vi "UI.vi"(8 "error in (no error)":errorcluster, 11 "View in":refnum<class "View.lvclass">) -> (0 "error out":errorcluster, 3 "View out":refnum<class "View.lvclass">)   [LabVIEW 2024, in "GUI.lvlib" / "View.lvclass"]
uses:
  View.lvclass
  Buttons/ButtonWhite.ctl
  Buttons/ButtonBlack.ctl
  Buttons/Key.ctl
  Buttons/Backspace.ctl
  Buttons/EnterKey.ctl
  TypeDefs/Yellow.ctl
  TypeDefs/Green.ctl
  TypeDefs/Grey.ctl
  TypeDefs/Red.ctl
  TypeDefs/White.ctl
  TypeDefs/LightGrey.ctl
  View.lvclass/View.ctl
panel:
  in  "Tab Control":enum32{"Home", "Settings", "Game", "Scores"}(tab)
  in  "Start Button":T1
  in  "Settings Button":T2
  in  "Back Button":T1
  in  "Difficulty":i32(slide)=1 min=1 max=5 step=1 scale=1.0..5.0
  in  "Guess Board":T3
  in  "Keyboard":T7
  in  "Home Button":T1
  in  "High Scores":i32(listbox)
  # "Easy"
  # "Hard"
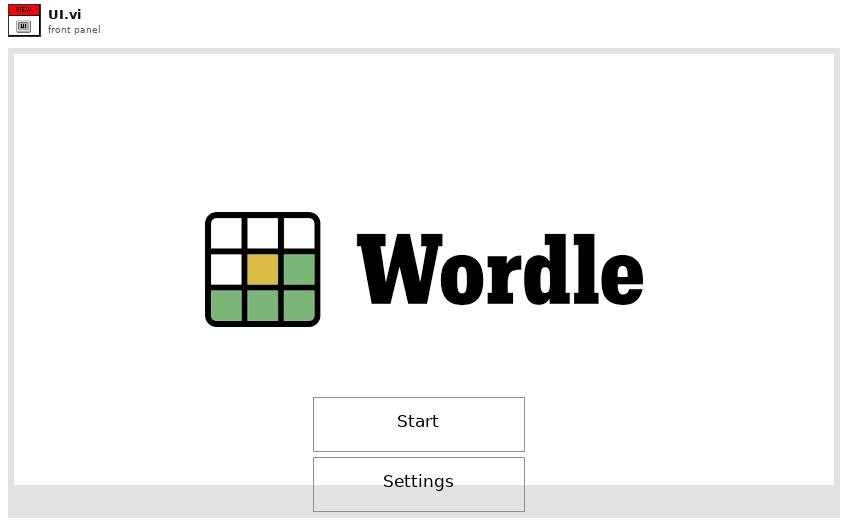
[diagram p1: front panel]
types:
  T1 = typedef "ButtonBlack.ctl" = bool
  T2 = typedef "ButtonWhite.ctl" = bool
  T3 = cluster{"Guess 1":cluster{"Letter 1":string, "Letter 2":string, "Letter 3":string, "Letter 4":string, "Letter 5":string}, "Guess 2":cluster{"Letter 1":string, "Letter 2":string, "Letter 3":string, "Letter 4":string, "Letter 5":string}, "Guess 3":cluster{"Letter 1":string, "Letter 2":string, "Letter 3":string, "Letter 4":string, "Letter 5":string}, "Guess 4":cluster{"Letter 1":string, "Letter 2":string, "Letter 3":string, "Letter 4":string, "Letter 5":string}, "Guess 5":cluster{"Letter 1":string, "Letter 2":string, "Letter 3":string, "Letter 4":string, "Letter 5":string}, "Guess 6":cluster{"Letter 1":string, "Letter 2":string, "Letter 3":string, "Letter 4":string, "Letter 5":string}}
  T4 = typedef "Key.ctl" = bool
  T5 = typedef "Backspace.ctl" = bool
  T6 = typedef "EnterKey.ctl" = bool
  T7 = cluster{"Q":T4, "W":T4, "E":T4, "R":T4, "T":T4, "Y":T4, "U":T4, "I":T4, "O":T4, "P":T4, "A":T4, "S":T4, "D":T4, "F":T4, "G":T4, "H":T4, "J":T4, "K":T4, "L":T4, "Z":T4, "X":T4, "C":T4, "V":T4, "B":T4, "N":T4, "M":T4, "Backspace":T5, "Enter":T6}
  T8 = typedef "LightGrey.ctl" = u32
  T9 = typedef "White.ctl" = u32
  T10 = typedef "Red.ctl" = u32
  T11 = typedef "Grey.ctl" = u32
  T12 = typedef "Green.ctl" = u32
  T13 = typedef "Yellow.ctl" = u32
  T14 = cluster{"This VI":refnum<vi>, "Tab Control":refnum<vi>, "Start Button":refnum<vi>, "Settings Button":refnum<vi>, "Back Button":refnum<vi>, "Difficulty":refnum<vi>, "Guess Board":refnum<vi>, "Keyboard":refnum<vi>, "High Scores":refnum<vi>, "Home Button":refnum<vi>}
  T15 = typedef "eventvkey.ctl" = enum16{"ASCII", "Enter", "Return", "Shift", "Ctrl", "Alt", "Cmd", "Opt", "Caps", "NumLock", "Clear", "Break", "Up", "Down", "Left", "Right", "Insert", "Delete", "Home", "End", "PageUp", "PageDown", "Escape", "Help", "Pause", "ScrollLock", "F1", "F2", "F3", "F4", "F5", "F6", "F7", "F8", "F9", "F10", "F11", "F12", "F13", "F14", "F15", "F16", "F17", "F18", "F19", "F20", "F21", "F22", "F23", "F24", "Play", "VolumeUp", "VolumeDown", "Mute", "Two Byte Char"}
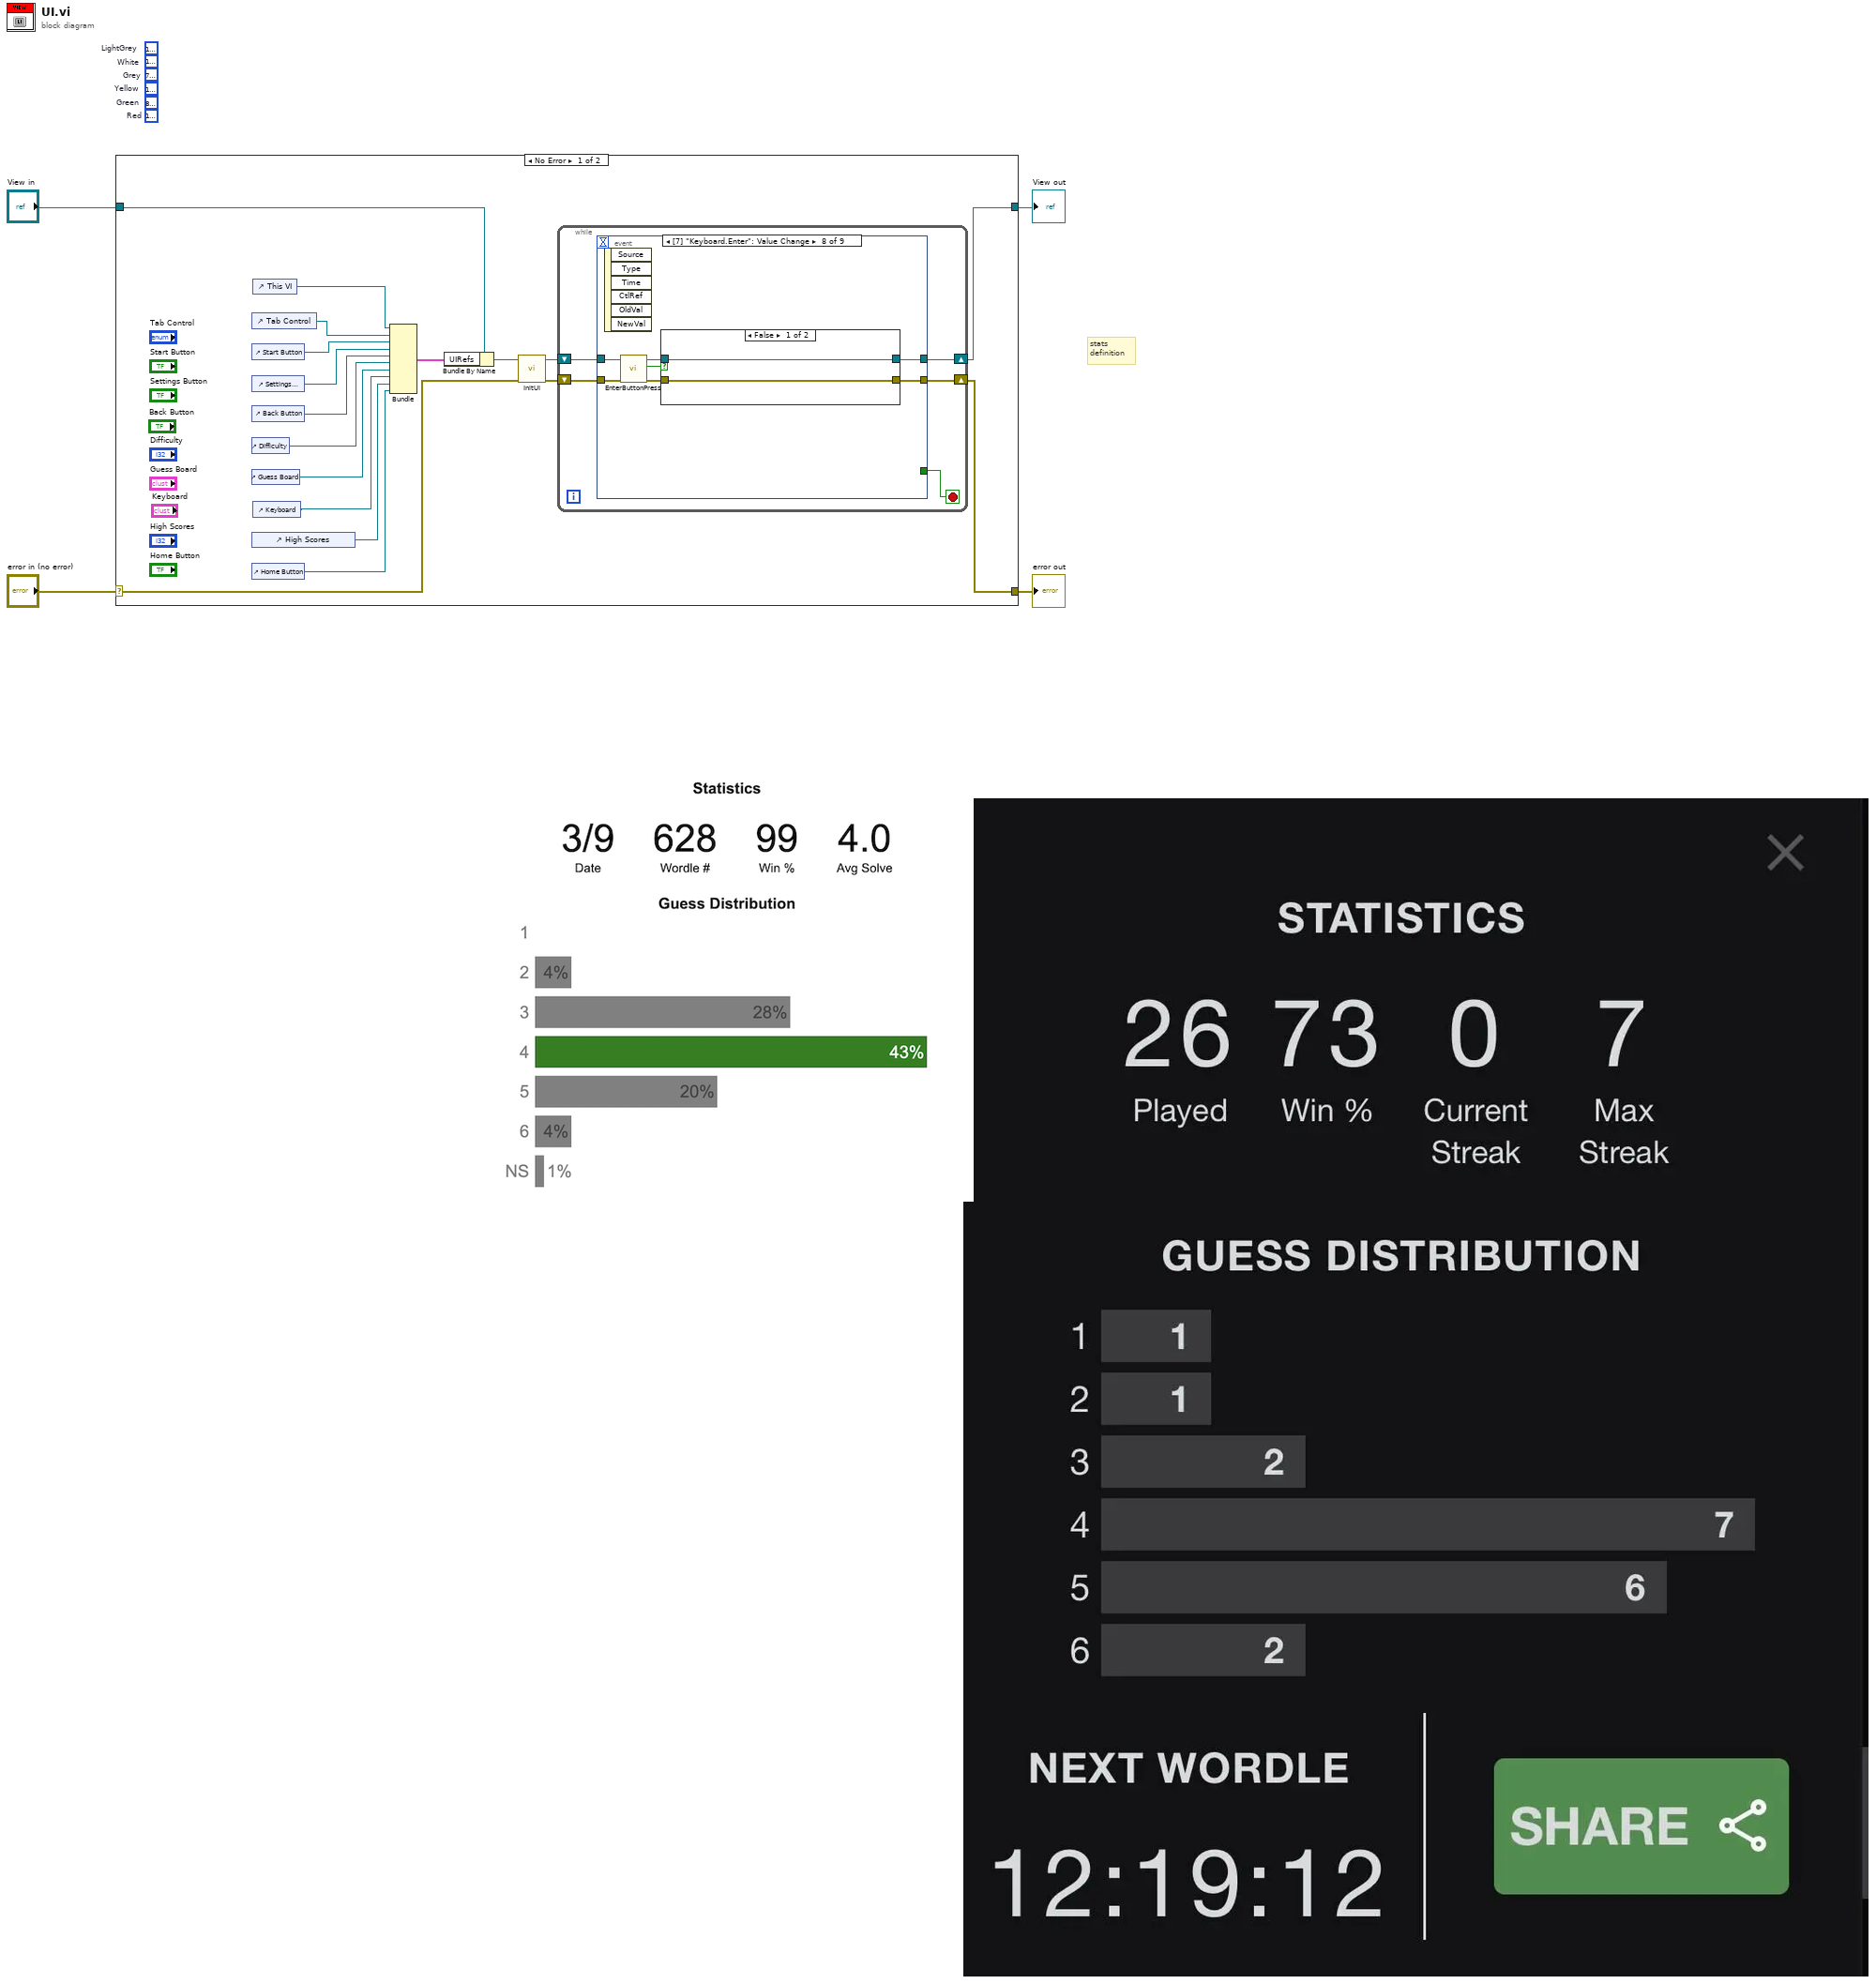
[diagram p0: block diagram]
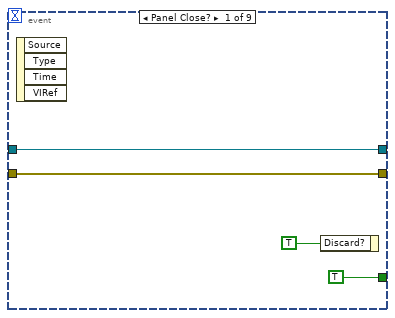
[diagram p2: hidden frame]
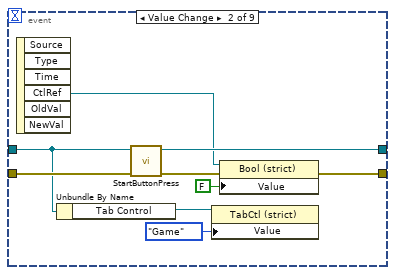
[diagram p3: hidden frame]
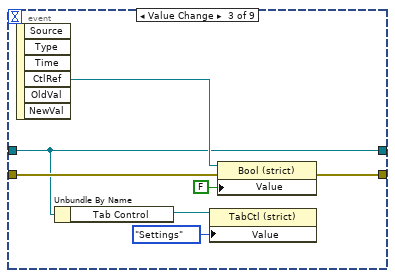
[diagram p4: hidden frame]
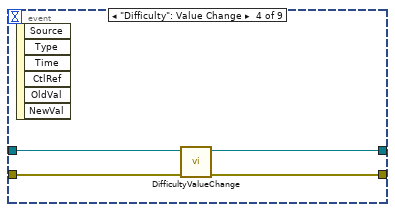
[diagram p5: hidden frame]
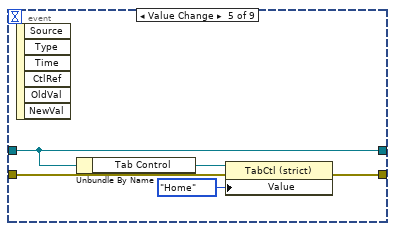
[diagram p6: hidden frame]
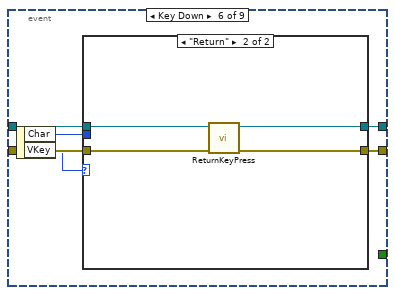
[diagram p7: hidden frame]
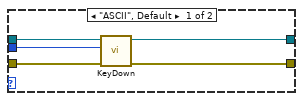
[diagram p8: hidden frame]
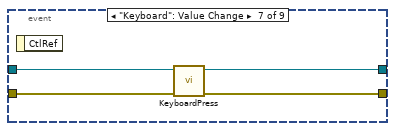
[diagram p9: hidden frame]
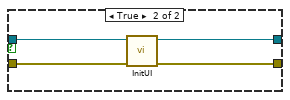
[diagram p10: hidden frame]
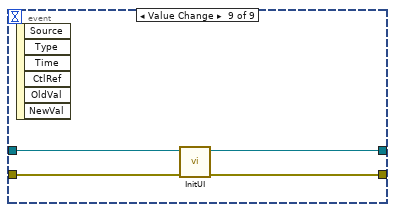
[diagram p11: hidden frame]
diagram:
  (unwired) T8 15461355  # LightGrey
  (unwired) T9 16777225  # White
  (unwired) T10 14425856  # Red
  (unwired) T11 7896190  # Grey
  (unwired) T12 8173175  # Green
  (unwired) T13 14400581  # Yellow
  # "stats\ndefinition"
  n1 = case shown="No Error" "error in (no error)" {
    selector: "error in (no error)" -> [w8 w94]
    tunnel: [w5 w94] -> w4
    tunnel: [w16 w93] -> w2
    tunnel: "View in" -> [w17 w93]
    frame No Error {
      n2 = control-ref of="Tab Control"() -> (w18:refnum<vi>)
      n3 = control-ref of="Start Button"() -> (w19:refnum<vi>)
      n4 = control-ref of="Settings Button"() -> (w20:refnum<vi>)
      n5 = control-ref of="Back Button"() -> (w11:refnum<vi>)
      n6 = control-ref of="Difficulty"() -> (w21:refnum<vi>)
      n7 = control-ref of="Guess Board"() -> (w15:refnum<vi>)
      n8 = control-ref of="High Scores"() -> (w22:refnum<vi>)
      n9 = control-ref of="Home Button"() -> (w14:refnum<vi>)
      n10 = control-ref of="This VI"() -> (w7:refnum<vi>)
      n11 = control-ref of="Keyboard"() -> (w10:refnum<vi>)
      n12 = Bundle("This VI"=w7, "Tab Control"=w18, "Start Button"=w19, "Settings Button"=w20, "Back Button"=w11, "Difficulty"=w21, "Guess Board"=w15, "Keyboard"=w10, "High Scores"=w22, "Home Button"=w14) -> (w9:T14)  [unwired: 1 in]
      n13 = Bundle By Name(cluster=w17, "UIRefs"=w9) -> (w13:refnum<class "View.lvclass">)
      n14 = call "InitUI.vi"("error in (no error)"=w8, "View in"=w13) -> ("error out"=w6:errorcluster, "View out"=w12:refnum<class "View.lvclass">)  [unwired: 8 in]
      n15 = while {
        shift-right: [w25] -> w5
        shift-left: w6 -> [w26]
        shift-right: [w23] -> w16
        shift-left: w12 -> [w24]
        stop <- w27 stop-if-true
        n16 = event shown="[7] \"Keyboard.Enter\": Value Change" {
          selector: _ -> [_ _ _ _ _ _ _ _ _]
          dyn-events: _ -> [_ _ _ _ _ _ _ _ _]
          timeout: _ -> [_ _ _ _ _ _ _ _ _]
          tunnel: [TRUE _ _ _ _ _ _ _ _] -> w27
          tunnel: w26 -> [w29 w40 w47 w50 w54 w59 w74 w81 w91]
          tunnel: [w29 w35 w45 w48 w55 w60 w72 w76 w89] -> w25
          tunnel: w24 -> [w28 w32 w41 w51 w53 w62 w75 w82 w92]
          tunnel: [w28 w39 w41 w49 w53 w61 w73 w77 w90] -> w23
          event Panel Close? {
            n17 = event-data() -> ()  [unwired: 1 in, 4 out]
            n18 = event-data("Discard?"=TRUE) -> ()  [unwired: 1 in, 1 out]
          }
          event Value Change {
            n19 = event-data() -> ("CtlRef"=w36:refnum<vi>)  [unwired: 1 in, 5 out]
            n20 = Unbundle By Name(w32) -> ("Tab Control"=w34:refnum<vi>)
            n21 = call "StartButtonPress.vi"("error in (no error)"=w40, "View in"=w32) -> ("error out"=w37:errorcluster, "View out"=w39:refnum<class "View.lvclass">)  [unwired: 8 in]
            n22 = property class="TabCtl (strict)"(reference=w34, "Value"=enum32{"Home", "Settings", "Game", "Scores"}."Game") -> ()  [unwired: 1 in, 2 out]
            n23 = property class="Bool (strict)"(reference=w36, error in=w37, "Value"=T2 FALSE) -> (error out=w35:errorcluster)  [unwired: 1 out]
          }
          event Value Change {
            n24 = event-data() -> ("CtlRef"=w46:refnum<vi>)  [unwired: 1 in, 5 out]
            n25 = Unbundle By Name(w41) -> ("Tab Control"=w43:refnum<vi>)
            n26 = property class="TabCtl (strict)"(reference=w43, "Value"=enum32{"Home", "Settings", "Game", "Scores"}."Settings") -> ()  [unwired: 1 in, 2 out]
            n27 = property class="Bool (strict)"(reference=w46, error in=w47, "Value"=T2 FALSE) -> (error out=w45:errorcluster)  [unwired: 1 out]
          }
          event "Difficulty": Value Change {
            n28 = event-data() -> ()  [unwired: 1 in, 6 out]
            n29 = call "DifficultyValueChange.vi"("error in (no error)"=w50, "View in"=w51) -> ("error out"=w48:errorcluster, "View out"=w49:refnum<class "View.lvclass">)  [unwired: 8 in]
          }
          event Value Change {
            n30 = event-data() -> ()  [unwired: 1 in, 6 out]
            n31 = Unbundle By Name(w53) -> ("Tab Control"=w56:refnum<vi>)
            n32 = property class="TabCtl (strict)"(reference=w56, error in=w54, "Value"=enum32{"Home", "Settings", "Game", "Scores"}."Home") -> (error out=w55:errorcluster)  [unwired: 1 out]
          }
          event Key Down {
            n33 = event-data() -> ("Char"=w58:i16, "VKey"=w57:T15)  [unwired: 1 in]
            n34 = case shown="\"Return\"" w57 {
              tunnel: w62 -> [w67 w71]
              tunnel: [w66 w68] -> w61
              tunnel: [w65 w69] -> w60
              tunnel: w59 -> [w64 w70]
              tunnel: w58 -> [w63 _]
              frame "ASCII", Default {
                n35 = call "KeyDown.vi"("error in (no error)"=w64, "Char"=w63, "View in"=w67) -> ("error out"=w65:errorcluster, "View out"=w66:refnum<class "View.lvclass">)  [unwired: 7 in]
              }
              frame "Return" {
                n36 = call "ReturnKeyPress.vi"("error in (no error)"=w70, "View in"=w71) -> ("error out"=w69:errorcluster, "View out"=w68:refnum<class "View.lvclass">)  [unwired: 8 in]
              }
            }
          }
          event "Keyboard": Value Change {
            n37 = event-data() -> ()  [unwired: 1 in, 1 out]
            n38 = call "KeyboardPress.vi"("error in (no error)"=w74, "View in"=w75) -> ("error out"=w72:errorcluster, "View out"=w73:refnum<class "View.lvclass">)  [unwired: 8 in]
          }
          event Value Change {
            n39 = event-data() -> ()  [unwired: 1 in, 6 out]
            n40 = call "EnterButtonPress.vi"("error in (no error)"=w81, "View in"=w82) -> ("error out"=w78:errorcluster, "endgame?"=w80:bool, "View out"=w79:refnum<class "View.lvclass">)  [unwired: 7 in]
            n41 = case shown="False" w80 {
              tunnel: w79 -> [w84 w88]
              tunnel: w78 -> [w83 w87]
              tunnel: [w84 w86] -> w77
              tunnel: [w83 w85] -> w76
              frame False {
              }
              frame True {
                n42 = call "InitUI.vi"("error in (no error)"=w87, "View in"=w88) -> ("error out"=w85:errorcluster, "View out"=w86:refnum<class "View.lvclass">)  [unwired: 8 in]
              }
            }
          }
          event Value Change {
            n43 = event-data() -> ()  [unwired: 1 in, 6 out]
            n44 = call "InitUI.vi"("error in (no error)"=w91, "View in"=w92) -> ("error out"=w89:errorcluster, "View out"=w90:refnum<class "View.lvclass">)  [unwired: 8 in]
          }
        }
      }
    }
    frame Error {
    }
  }
  "error out" <- w4
  "View out" <- w2
